vi "Labview6_2.vi"() -> ()   [LabVIEW 2016]
panel:
  out "Numeric":dbl
  in  "stop":bool
  out "Boolean 2":bool
  out "Small Cluster":cluster{"Boolean":bool, "Slide Value":dbl}
  out "Modified Cluster":T1 {"Slide" scale=0.0..10.0}
  in  "Cluster":T1 {"Slide" scale=0.0..10.0}
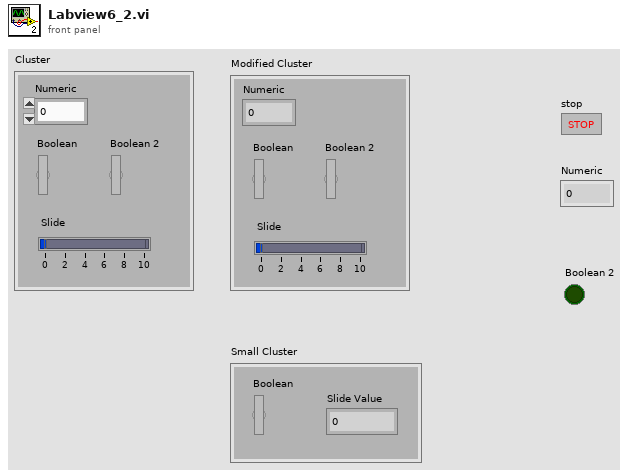
[diagram p1: front panel]
types:
  T1 = cluster{"Numeric":dbl, "Boolean":bool, "Boolean 2":bool, "Slide":dbl}
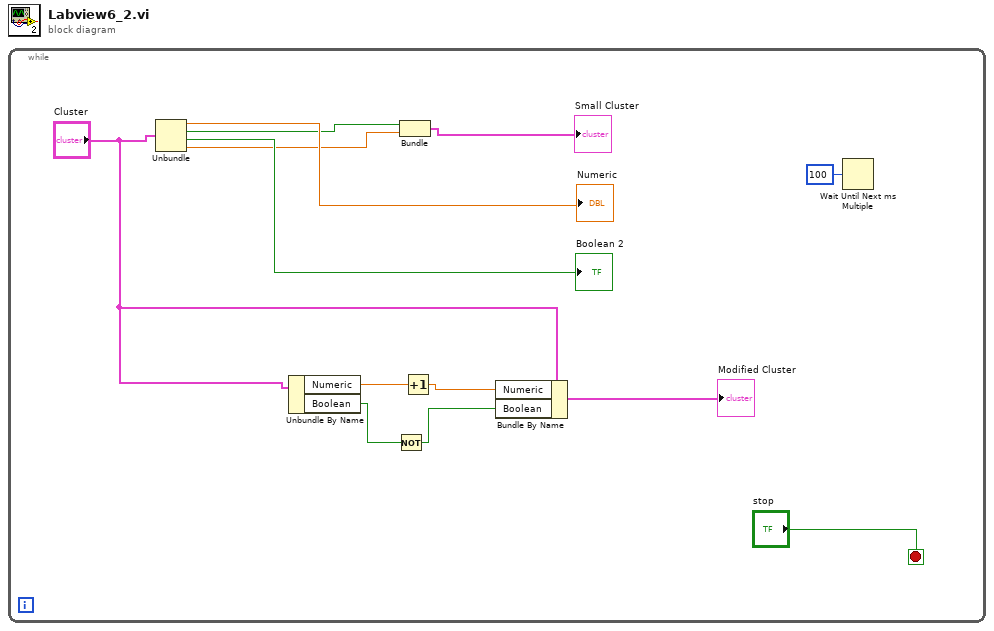
[diagram p0: block diagram]
diagram:
  n1 = while {
    stop <- "stop" stop-if-true
    n2 = Unbundle "Unbundle"("Cluster") -> ("Numeric"=→"Numeric":dbl, "Boolean"=w10:bool, "Boolean 2"=→"Boolean 2":bool, "Slide"=w9:dbl)
    n3 = Unbundle By Name "Unbundle By Name"("Cluster") -> ("Numeric"=w6:dbl, "Boolean"=w7:bool)
    n4 = Not(x=w7) -> (.not. x?=w4:bool)
    n5 = Bundle "Bundle"("Boolean"=w10, "Slide"=w9) -> (→"Small Cluster":cluster{"Boolean":bool, "Slide":dbl})  [unwired: 1 in]
    n6 = Increment(x=w6) -> (x+1=w5:dbl)
    n7 = Bundle By Name(cluster="Cluster", "Numeric"=w5, "Boolean"=w4) -> (→"Modified Cluster":T1)
    n8 = Wait Until Next ms Multiple(millisecond multiple=u32 100) -> ()  [unwired: 1 out]
  }
